vi "ONeilAxialP.vi"(1 "Trans Geometry":T1={"Radius (cm)"=9.0, "a (cm)"=4.0, "focus location"=9.0} {"focus location" format="%.2f"; "a (cm)" format="%.2f"; "Radius (cm)" format="%.2f"}, 2 "Variables":T2={"Number of rings"=8, "sound spd (cm/s)"=150000, "z span (cm)"=4.0, "z steps"=80, "y span (cm)"=0.1, "y steps"=10, "time step (s)"=1e-09, "z"=0.0, "y"=0.0, "ref delay"=0.0, "freq (MHz)"=4.5, "cycles"=5} {"freq (MHz)" format="%.2f"; "z span (cm)" format="%.2f"; "y" format="%.2f"; "ref delay" format="%.2f"; "y span (cm)" format="%.3f"; "z" format="%.2f"; "time step (s)" format="%.2e"}) -> (0 "Output Variable":dbl format="%.2f")   [LabVIEW 2022 SP3]
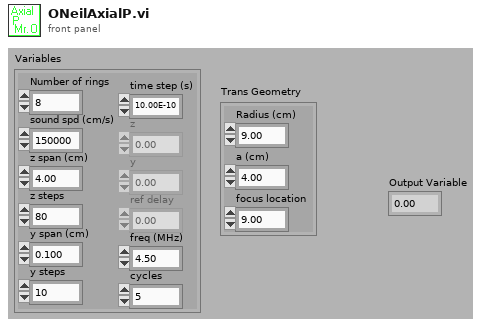
[diagram p1: front panel]
types:
  T1 = cluster{"Radius (cm)":dbl, "a (cm)":dbl, "focus location":dbl}
  T2 = cluster{"Number of rings":i32, "sound spd (cm/s)":i32, "z span (cm)":dbl, "z steps":i32, "y span (cm)":dbl, "y steps":i32, "time step (s)":sgl, "z":dbl, "y":dbl, "ref delay":dbl, "freq (MHz)":dbl, "cycles":i32}
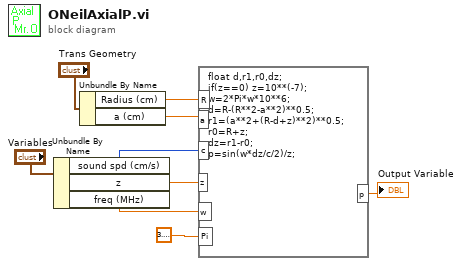
[diagram p0: block diagram]
diagram:
  n1 = Unbundle By Name("Variables") -> ("sound spd (cm/s)"=w4:i32, "z"=w8:dbl, "freq (MHz)"=w2:dbl)
  n2 = Unbundle By Name("Trans Geometry") -> ("Radius (cm)"=w6:dbl, "a (cm)"=w5:dbl)
  n3 = formula code="float d,r1,r0,dz;\nif(z==0) z=10**(-7);\nw=2*Pi*w*10**6;\nd=R-(R**2-a**2)**0.5;\nr1=(a**2+(R-d+z)**2)**0.5;\nr0=R+z;\ndz=r1-r0;\np=sin(w*dz/c/2)/z;"("a"=w5, "R"=w6, "z"=w8, "c"=w4, "w"=w2, "Pi"=3.141592653589793) -> ("p"=→"Output Variable":dbl)
